vi "Local Variables.vi"() -> ()   [LabVIEW 2009]
panel:
  in  "Contrôle des boucles":bool
  out "Graphe déroulant 2":dbl(graph)
  out "Graphe déroulant 1":dbl(graph)
  # "Off"
  # "On"
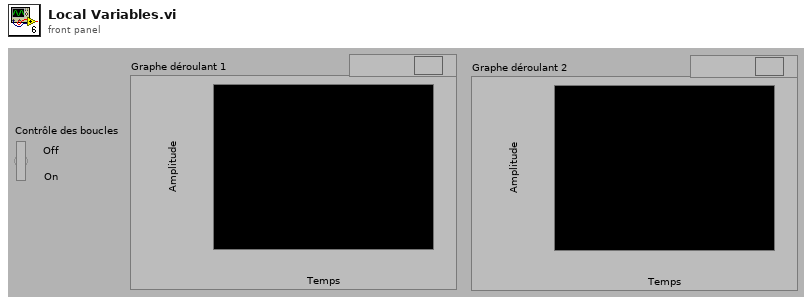
[diagram p1: front panel]
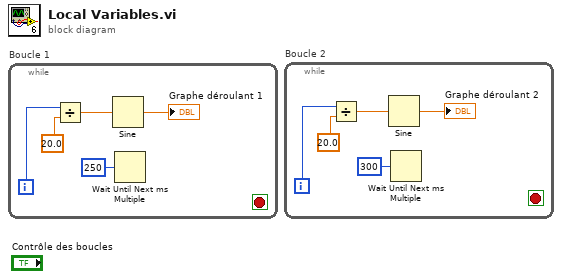
[diagram p0: block diagram]
diagram:
  n1 = while "Boucle 1" {
    i -> [w5]
    stop <- _ stop-if-true
    n2 = Divide ("Diviser")(x=w5, y=20.0) -> (x/y=w3:dbl)
    n3 = Sine ("Sinus")(x=w3) -> (sin(x)=→"Graphe déroulant 1":dbl)
    n4 = Wait Until Next ms Multiple ("Attendre un multiple de ms")(millisecond multiple=u32 250) -> ()  [unwired: 1 out]
  }
  n5 = while "Boucle 2" {
    i -> [w10]
    stop <- _ stop-if-true
    n6 = Divide ("Diviser")(x=w10, y=20.0) -> (x/y=w8:dbl)
    n7 = Sine ("Sinus")(x=w8) -> (sin(x)=→"Graphe déroulant 2":dbl)
    n8 = Wait Until Next ms Multiple ("Attendre un multiple de ms")(millisecond multiple=u32 300) -> ()  [unwired: 1 out]
  }
